vi "LCD_SET_COLOR.vi"(11 "String in":string) -> (3 "String out":string)   [LabVIEW 2015]
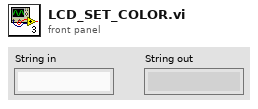
[diagram p1: front panel]
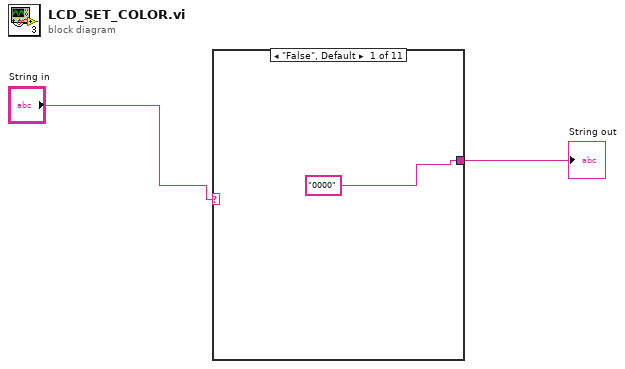
[diagram p0: block diagram]
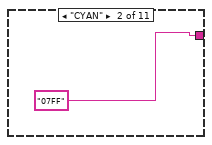
[diagram p2: hidden frame]
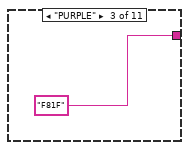
[diagram p3: hidden frame]
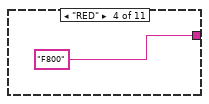
[diagram p4: hidden frame]
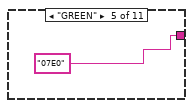
[diagram p5: hidden frame]
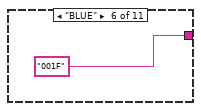
[diagram p6: hidden frame]
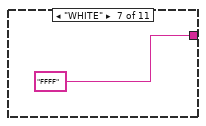
[diagram p7: hidden frame]
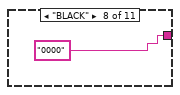
[diagram p8: hidden frame]
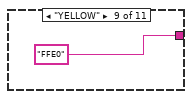
[diagram p9: hidden frame]
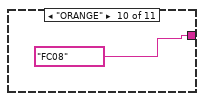
[diagram p10: hidden frame]
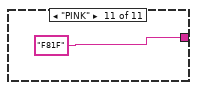
[diagram p11: hidden frame]
diagram:
  n1 = case shown="\"False\", Default" "String in" {
    tunnel: ["0000" "07FF" "F81F" "F800" "07E0" "001F" "FFFF" "0000" "FFE0" "FC08" "F81F"] -> w2
    frame "False", Default {
    }
    frame "CYAN" {
    }
    frame "PURPLE" {
    }
    frame "RED" {
    }
    frame "GREEN" {
    }
    frame "BLUE" {
    }
    frame "WHITE" {
    }
    frame "BLACK" {
    }
    frame "YELLOW" {
    }
    frame "ORANGE" {
    }
    frame "PINK" {
    }
  }
  "String out" <- w2
